vi "Get Best Case Error.vi"(4 "error 2 in (no error)":errorcluster, 5 "error 1 in (no error)":errorcluster) -> (0 "error out":errorcluster)   [LabVIEW 2021, in "Error.lvlib"]
uses:
  Error.lvlib
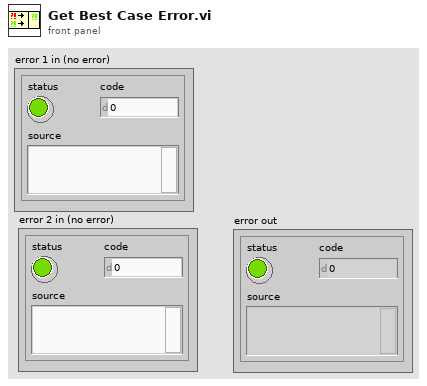
[diagram p1: front panel]
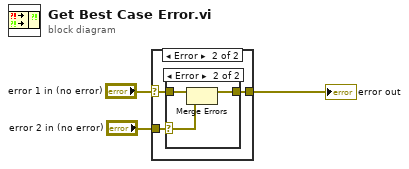
[diagram p0: block diagram]
diagram:
  n1 = case shown="Error" "error 1 in (no error)" {
    selector: "error 1 in (no error)" -> [w4 w5]
    tunnel: "error 2 in (no error)" -> [_ w7]
    tunnel: [w4 w6] -> w1
    frame No Error {
    }
    frame Error {
      n2 = case shown="Error" w7 {
        selector: w7 -> [w8 w10]
        tunnel: [w8 w9] -> w6
        tunnel: w5 -> [_ w11]
        frame No Error {
        }
        frame Error {
          n3 = Merge Errors(w11, w10) -> (w9:errorcluster)
        }
      }
    }
  }
  "error out" <- w1
